vi "flag_write.vi"(5 "flag number":i32, 9 "flag value":bool, 11 "error in (no error)":errorcluster) -> (15 "error out":errorcluster)   [LabVIEW 2016]
uses:
  flag_array.vi
panel:
  out "Array":bool[](array[boolean])
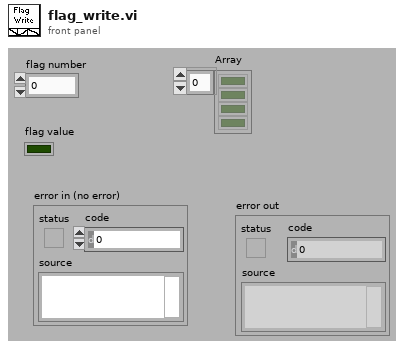
[diagram p1: front panel]
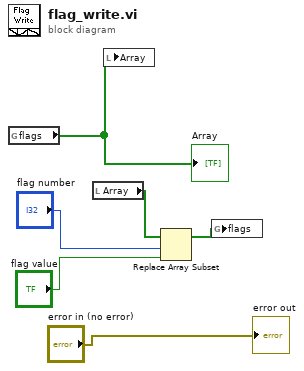
[diagram p0: block diagram]
diagram:
  n1 = global read "flag_array.vi" "flags"() -> (w2:bool[])
  "Array" <- w2
  n2 = local read "Array"() -> (w1:bool[])
  n3 = local write "Array"(w2) -> ()
  n4 = Replace Array Subset(array=w1, new element="flag value", index="flag number") -> (w4:bool[])
  n5 = global write "flag_array.vi" "flags"(w4) -> ()
  "error out" <- "error in (no error)"
